vi "Next API Number.vi"(11 "VolatusCore in":refnum<class "VolatusCore.lvclass">) -> (2 "Next API":u32, 3 "VolatusCore out":refnum<class "VolatusCore.lvclass">)   [LabVIEW 2020, in "Volatus.lvlib" / "VolatusCore.lvclass"]
uses:
  VolatusCore.lvclass
  VolatusCore.lvclass/VolatusCore.ctl
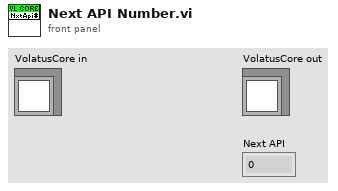
[diagram p1: front panel]
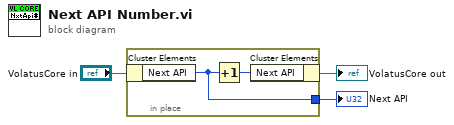
[diagram p0: block diagram]
diagram:
  n1 = in-place {
    in-place-border: [w4] -> w2
    n2 = in-place-cluster #1("VolatusCore in") -> ("Next API"=w4:u32)
    n3 = Increment(x=w4) -> (x+1=w5:u32)
    n4 = in-place-cluster #1("Next API"=w5) -> (→"VolatusCore out":refnum<class "VolatusCore.lvclass">)
  }
  "Next API" <- w2
